vi "Func-엑셀 데이터를 그래프로 출력.vi"() -> ()   [LabVIEW 2015] (continued)
\n85\t85\t83.883\n85\t85\t83.891\n85\t85\t83.897\n85\t85\t83.907\n85\t85\t83.917\n85\t85\t83.924\n85\t85\t83.937\n85\t85\t83.942\n85\t85\t83.946\n85\t85\t83.956\n85\t85\t83.957\n85\t85.01\t83.959\n85\t85.01\t83.961\n85\t85.01\t83.965\n85\t85.01\t83.97\n85\t85.01\t83.974\n85\t85.01\t83.984\n85\t85.01\t83.996\n85\t85.01\t84\n85\t85.01\t84.004\n85\t85.01\t84.016\n85\t85.01\t84.023\n85\t85.01\t84.028\n85\t85.01\t84.036\n85\t85.01\t84.041\n85\t85.01\t84.044\n85\t85.01\t84.05\n85\t85.01\t84.058\n85\t85.01\t84.063\n85\t85.01\t84.074\n85\t85.01\t84.08\n85\t85.01\t84.095\n85\t85.01\t84.101\n85\t85.01\t84.103\n85\t85.01\t84.113\n85\t85.01\t84.116\n85\t85.01\t84.121\n85\t85.01\t84.126\n85\t85.01\t84.13\n85\t85.01\t84.139\n85\t85.01\t84.14\n85\t85.01\t84.146\n85\t85.01\t84.151\n85\t85.01\t84.157\n85\t85.01\t84.165\n85\t85.01\t84.17\n85\t85.01\t84.18\n85\t85.01\t84.185\n85\t85.01\t84.195\n85\t85.01\t84.2\n85\t85.01\t84.202\n85\t85.01\t84.207\n85\t85.01\t84.211\n85\t85.01\t84.218\n85\t85.01\t84.225\n85\t85.01\t84.23\n85\t85.01\t84.238\n85\t85.01\t84.242\n85\t85.01\t84.247\n85\t85.01\t84.253\n85\t85.01\t84.257\n85\t85.01\t84.261\n85\t85.01\t84.266\n85\t85.01\t84.273\n85\t85.01\t84.276\n85\t85.01\t84.28\n85\t85.01\t84.286\n85\t85.01\t84.292\n85\t85.01\t84.3\n85\t85.01\t84.303\n85\t85.01\t84.312\n85\t85.01\t84.321\n85\t85.01\t84.327\n85\t85.01\t84.332\n85\t85\t84.339\n85\t85\t84.35\n85\t85\t84.354\n85\t85\t84.359\n85\t85\t84.36\n85\t85\t84.367\n85\t85\t84.372\n85\t85\t84.376\n85\t85\t84.385\n85\t85\t84.395\n85\t85\t84.406\n85\t85\t84.411\n85\t85\t84.419\n85\t85\t84.423\n85\t85\t84.432\n85\t85\t84.433\n85\t85\t84.438\n85\t85\t84.446\n85\t85\t84.448\n85\t85\t84.454\n85\t85\t84.46\n85\t85\t84.464\n85\t85\t84.47\n85\t85\t84.474\n85\t85\t84.48\n85\t85\t84.484\n85\t85\t84.487\n85\t85\t84.494\n85\t85\t84.5\n85\t85\t84.507\n85\t85\t84.516\n85\t85\t84.524\n85\t85\t84.53\n85\t85\t84.536\n85\t85\t84.544\n85\t85\t84.547\n85\t85\t84.552\n85\t85\t84.556\n85\t85\t84.564\n85\t85\t84.569\n85\t85\t84.575\n85\t85\t84.582\n85\t85\t84.59\n85\t85\t84.595\n85\t85\t84.595\n85\t85\t84.602\n85\t85\t84.605\n85\t85\t84.61\n85\t85\t84.614\n85\t85\t84.62\n85\t85\t84.626\n85\t85\t84.634\n85\t85\t84.636\n85\t85\t84.64\n85\t85\t84.642\n85\t85\t84.648\n85\t85\t84.658\n85\t85\t84.659\n85\t85\t84.665\n85\t85\t84.671\n85\t85\t84.679\n85\t85\t84.684\n85\t85\t84.692\n85\t85\t84.699\n85\t85\t84.705\n85\t85\t84.715\n85\t85\t84.715\n85\t85\t84.72\n85\t85\t84.729\n85\t85\t84.736\n85\t85\t84.745\n85\t85\t84.751\n85\t85\t84.759\n85\t85\t84.764\n85\t85\t84.769\n85\t85\t84.773\n85\t85\t84.782\n85\t85\t84.787\n85\t85\t84.791\n85\t85\t84.804\n85\t85\t84.804\n85\t85\t84.81\n85\t85\t84.812\n85\t85\t84.818\n85\t85\t84.823\n85\t85\t84.823\n85\t85\t84.83\n85\t85\t84.833\n85\t85\t84.84\n85\t85\t84.846\n85\t85\t84.854\n85\t85\t84.863\n85\t85\t84.866\n85\t85\t84.872\n85\t85\t84.878\n85\t85\t84.879\n85\t85\t84.884\n85\t85\t84.886\n85\t85\t84.891\n85\t85\t84.902\n85\t85\t84.904\n85\t85\t84.91\n85\t85\t84.92\n85\t85\t84.922\n85\t85\t84.927\n85\t85\t84.932\n85\t85\t84.939\n85\t85\t84.946\n85\t85\t84.948\n85\t85\t84.953\n85\t85\t84.961\n85\t85\t84.965\n85\t85\t84.969\n85\t85\t84.973\n85\t85\t84.979\n85\t85\t84.987\n85\t85\t84.993\n85\t85\t84.996\n85\t85\t85.003\n85\t85\t85.014\n85\t85\t85.018\n85\t85\t85.023\n85\t85\t85.032\n85\t85\t85.036\n85\t85\t85.043\n85\t85\t85.048\n85\t85\t85.053\n85\t85\t85.059\n85\t85\t85.062\n85\t85\t85.067\n85\t85\t85.068\n85\t85\t85.069\n85\t85\t85.072\n85\t85\t85.075\n85\t85\t85.079\n85\t85\t85.083\n85\t85\t85.089\n85\t85\t85.096\n85\t85\t85.104\n85\t85\t85.11\n85\t85\t85.117\n85\t85\t85.128\n85\t85\t85.136\n85\t85\t85.14\n85\t85\t85.146\n85\t85\t85.153\n85\t85\t85.155\n85\t85\t85.156\n85\t85\t85.159\n85\t85\t85.163\n85\t85\t85.169\n85\t85\t85.171\n85\t85\t85.175\n85\t85\t85.185\n85\t85\t85.189\n85\t85\t85.196\n85\t85\t85.198\n85\t85\t85.203\n85\t85\t85.21\n85\t85\t85.216\n85\t85\t85.22\n85\t85\t85.227\n85\t85\t85.238\n85\t85\t85.244\n85\t85\t85.251\n85\t85\t85.253\n85\t85\t85.257\n85\t85\t85.261\n85\t85\t85.262\n85\t85\t85.263\n85\t85\t85.268\n85\t85\t85.271\n85\t85\t85.277\n85\t85\t85.283\n85\t85\t85.287\n85\t85\t85.297\n85\t85\t85.297\n85\t85\t85.302\n85\t85\t85.309\n85\t85\t85.316\n85\t85\t85.324\n85\t85\t85.333\n85\t85\t85.343\n85\t85\t85.35\n85\t85\t85.356\n85\t85\t85.36\n85\t85\t85.367\n85\t85\t85.37\n85\t85\t85.372\n85\t85\t85.375\n85\t85\t85.377\n85\t85\t85.383\n85\t85\t85.382\n85\t85\t85.384\n85\t85\t85.384\n85\t85\t85.395\n85\t85\t85.4\n85\t85\t85.401\n85\t85\t85.408\n85\t85\t85.414\n85\t85\t85.42\n85\t85\t85.424\n85\t85\t85.432\n85\t85\t85.438\n85\t85\t85.446\n85\t85\t85.451\n85\t85\t85.455\n85\t85\t85.459\n85\t85\t85.464\n85\t85\t85.471\n85\t85\t85.48\n85\t85\t85.484\n85\t85\t85.493\n85\t85\t85.495\n85\t85\t85.495\n85\t85\t85.499\n85\t85\t85.5\n85\t85\t85.502\n85\t85\t85.508\n85\t85\t85.516\n85\t85\t85.527\n85\t85\t85.537\n85\t85\t85.542\n85\t85\t85.548\n85\t85\t85.552\n85\t85\t85.552\n85\t85\t85.555\n85\t85\t85.557\n85\t85\t85.563\n85\t85\t85.568\n85\t85\t85.573\n85\t85\t85.58\n85\t85\t85.583\n85\t85\t85.588\n85\t85\t85.591\n85\t85\t85.598\n85\t85\t85.604\n85\t85\t85.609\n85\t85\t85.616\n85\t85\t85.62\n85\t85\t85.622\n85\t85\t85.625\n85\t85\t85.632\n85\t85\t85.634\n85\t85\t85.634\n85\t85\t85.639\n85\t85\t85.643\n85\t85\t85.647\n85\t85\t85.648\n85\t85\t85.657\n85\t85\t85.666\n85\t85\t85.668\n85\t85\t85.675\n85\t85\t85.682\n85\t85\t85.685\n85\t85\t85.686\n85\t85\t85.688\n85\t85\t85.693\n85\t85\t85.7\n85\t85\t85.703\n85\t85\t85.715\n85\t85\t85.721\n85\t85\t85.724\n85\t85\t85.732\n85\t85\t85.734\n85\t85\t85.736\n85\t85\t85.738\n85\t85\t85.743\n85\t85\t85.753\n85\t85\t85.758\n85\t85\t85.762\n85\t85\t85.764\n85\t85\t85.769\n85\t85\t85.771\n85\t85\t85.774\n85\t85\t85.775\n85\t85\t85.783\n85\t85\t85.798\n85\t85\t85.802\n85\t85\t85.807\n85\t85\t85.812\n85\t85\t85.816\n85\t85\t85.819\n85\t85\t85.816\n85\t85\t85.821\n85\t85\t85.829\n85\t85\t85.833\n85\t85\t85.834\n85\t85\t85.839\n85\t85\t85.848\n85\t85\t85.853\n85\t85\t85.854\n85\t85\t85.858\n85\t85\t85.868\n85\t85\t85.871\n85\t85\t85.872\n85\t85\t85.874\n85\t85\t85.885\n85\t85\t85.89\n85\t85\t85.895\n85\t85\t85.9\n85\t85\t85.904\n85\t85\t85.909\n85\t85\t85.912\n85\t85\t85.916\n85\t85\t85.918\n85\t85\t85.925\n85\t85\t85.93\n85\t85\t85.938\n85\t85\t85.942\n85\t85\t85.944\n85\t85\t85.953\n85\t85\t85.953\n85\t85\t85.955\n85\t85\t85.96\n85\t85\t85.964\n85\t85\t85.965\n85\t85\t85.973\n85\t85\t85.978\n85\t85\t85.98\n85\t85\t85.983\n85\t85\t85.986\n85\t85\t85.991\n85\t85\t85.994\n85\t85\t85.995\n85\t85\t86.002\n85\t85\t86.005\n85\t85\t86.012\n85\t85\t86.02\n85\t85\t86.024\n85\t85\t86.028\n85\t85\t86.03\n85\t85\t86.032\n85\t85\t86.037\n85\t85\t86.039\n85\t85\t86.04\n85\t85\t86.046\n85\t85\t86.049\n85\t85\t86.054\n85\t85\t86.058\n85\t85\t86.061\n85\t85\t86.066\n85\t85\t86.072\n85\t85\t86.079\n85\t85\t86.087\n85\t85\t86.091\n85\t85\t86.096\n85\t85\t86.098\n85\t85\t86.102\n85\t85\t86.109\n85\t85\t86.113\n85\t85\t86.118\n85\t85\t86.117\n85\t85\t86.122\n85\t85\t86.123\n85\t85\t86.128\n85\t85\t86.134\n85\t85\t86.138\n85\t85\t86.146\n85\t85\t86.151\n85\t85\t86.159\n85\t85\t86.159\n85\t85\t86.166\n85\t85\t86.167\n85\t85\t86.171\n85\t85.01\t86.178\n85\t85.01\t86.176\n85\t85.01\t86.182\n85\t85.01\t86.187\n85\t85.01\t86.193\n85\t85.01\t86.196\n85\t85.01\t86.2\n85\t85.01\t86.205\n85\t85.01\t86.204\n85\t85.01\t86.208\n85\t85.01\t86.214\n85\t85.01\t86.222\n85\t85.01\t86.227\n85\t85.01\t86.232\n85\t85.01\t86.236\n85\t85.01\t86.239\n85\t85.01\t86.239\n85\t85.01\t86.24\n85\t85.01\t86.238\n85\t85.01\t86.245\n85\t85.01\t86.249\n85\t85.01\t86.252\n85\t85.01\t86.253\n85\t85.01\t86.259\n85\t85.01\t86.266\n85\t85.01\t86.27\n85\t85.01\t86.275\n85\t85.01\t86.279\n85\t85.01\t86.287\n85\t85.01\t86.289\n85\t85.01\t86.29\n85\t85.01\t86.293\n85\t85.01\t86.293\n85\t85.01\t86.301\n85\t85.01\t86.304\n85\t85.01\t86.308\n85\t85.01\t86.317\n85\t85.01\t86.326\n85\t85.01\t86.328\n85\t85.01\t86.331\n85\t85.01\t86.334\n85\t85.01\t86.34\n85\t85.01\t86.342\n85\t85.01\t86.343\n85\t85.01\t86.349\n85\t85.01\t86.355\n85\t85.01\t86.36\n85\t85\t86.364\n85\t85\t86.37\n85\t85.01\t86.373\n85\t85.01\t86.379\n85\t85.01\t86.382\n85\t85.01\t86.383\n85\t85.01\t86.389\n85\t85.01\t86.393\n85\t85\t86.398\n85\t85.01\t86.404\n85\t85.01\t86.407\n85\t85.01\t86.411\n85\t85.01\t86.413\n85\t85.01\t86.411\n85\t85.01\t86.412\n85\t85.01\t86.416\n85\t85\t86.419\n85\t85\t86.423\n85\t85\t86.429\n85\t85\t86.436\n85\t85\t86.438\n85\t85\t86.441\n85\t85\t86.445\n85\t85\t86.448\n85\t85\t86.452\n85\t85\t86.458\n85\t85\t86.469\n85\t85\t86.472\n85\t85\t86.477\n85\t85\t86.484\n85\t85\t86.484\n85\t85\t86.485\n85\t85\t86.487\n85\t85\t86.489\n85\t85\t86.495\n85\t85\t86.499\n85\t85\t86.501\n85\t85\t86.501\n85\t85\t86.504\n85\t85\t86.507\n85\t85\t86.512\n85\t85\t86.516\n85\t85\t86.523\n85\t85\t86.531\n85\t85\t86.536\n85\t85\t86.54\n85\t85\t86.545\n85\t85\t86.549\n85\t85\t86.55\n85\t85\t86.556\n85\t85\t86.561\n85\t85\t86.565\n85\t85\t86.566\n85\t85\t86.568\n85\t85\t86.575\n85\t85\t86.575\n85\t85\t86.579\n85\t85\t86.583\n85\t85\t86.588\n85\t85\t86.593\n85\t85\t86.595\n85\t85\t86.601\n85\t85\t86.604\n85\t85\t86.609\n85\t85\t86.611\n85\t85\t86.618\n85\t85\t86.623\n85\t85\t86.628\n85\t85\t86.629\n85\t85\t86.635\n85\t85\t86.639\n85\t85\t86.637\n85\t85\t86.637\n85\t85\t86.638\n85\t85\t86.641\n85\t85\t86.643\n85\t85\t86.647\n85\t85\t86.651\n85\t85\t86.656\n85\t85\t86.658\n85\t85\t86.665\n85\t85\t86.669\n85\t85\t86.677\n85\t85\t86.682\n85\t85\t86.683\n85\t85\t86.689\n85\t85\t86.693\n85\t85\t86.694\n85\t85\t86.694\n85\t85\t86.695\n85\t85\t86.699\n85\t85\t86.702\n85\t85\t86.705\n85\t85\t86.71\n85\t85\t86.713\n85\t85\t86.714\n85\t85\t86.72\n85\t85\t86.722\n85\t85\t86.727\n85\t85\t86.729\n85\t85\t86.739\n85\t85\t86.746\n85\t85\t86.75\n85\t85\t86.755\n85\t85\t86.757\n85\t85\t86.761\n85\t85\t86.766\n85\t85\t86.765\n85\t85\t86.772\n85\t85\t86.774\n85\t85\t86.775\n85\t85\t86.781\n85\t85\t86.78\n85\t85\t86.789\n85\t85\t86.79\n85\t85\t86.793\n85\t85\t86.799\n85\t85\t86.803\n85\t85\t86.805\n85\t85\t86.806\n85\t85\t86.809\n85\t85\t86.813\n85\t85\t86.816\n85\t85\t86.816\n85\t85\t86.818\n85\t85\t86.821\n85\t85\t86.825\n85\t85\t86.825\n85\t85\t86.832\n85\t85\t86.836\n85\t85\t86.842\n85\t85\t86.85\n85\t85\t86.851\n85\t85\t86.855\n85\t85\t86.854\n85\t85\t86.855\n85\t85\t86.859\n85\t85\t86.859\n85\t85\t86.865\n85\t85\t86.873\n85\t85\t86.878\n85\t85\t86.882\n85\t85\t86.887\n85\t85\t86.889\n85\t85\t86.892\n85\t85\t86.892\n85\t85\t86.893\n85\t85\t86.9\n85\t85\t86.902\n85\t85\t86.907\n85\t85\t86.907\n85\t85\t86.909\n85\t85\t86.912\n85\t85\t86.915\n85\t85\t86.917\n85\t85\t86.919\n85\t85\t86.922\n85\t85\t86.925\n85\t85\t86.933\n85\t85\t86.937\n85\t85\t86.941\n85\t85\t86.941\n85\t85\t86.953\n85\t85\t86.956\n85\t85\t86.954\n85\t85\t86.961\n85\t85\t86.964\n85\t85\t86.965\n85\t85\t86.963\n85\t85\t86.968\n85\t85\t86.973\n85\t85\t86.977\n85\t85\t86.976\n85\t85\t86.984\n85\t85\t86.988\n85\t85\t86.993\n85\t85\t86.999\n85\t85\t86.997\n85\t85\t87.004\n85\t85\t87.005\n85\t85\t87.007\n85\t85\t87.008\n85\t85\t87.013\n85\t85\t87.017\n85\t85\t87.022\n85\t85\t87.027\n85\t85\t87.029\n85\t85\t87.029\n85\t85\t87.032\n85\t85\t87.037\n85\t85\t87.041\n85\t85\t87.044\n85\t85\t87.048\n85\t85\t87.055\n85\t85\t87.058\n85\t85\t87.058\n85\t85\t87.059\n85\t85\t87.059\n85\t85\t87.065\n85\t85\t87.069\n85\t85\t87.073\n85\t85\t87.078\n85\t85\t87.085\n85\t85\t87.09\n85\t85\t87.088\n85\t85\t87.089\n85\t85\t87.091\n85\t85\t87.098\n85\t85\t87.101\n85\t85\t87.1\n85\t85\t87.106\n85\t85\t87.107\n85\t85\t87.11\n85\t85\t87.111\n85\t85\t87.112\n85\t85\t87.115\n85\t85\t87.121\n85\t85\t87.123\n85\t85\t87.128\n85\t85\t87.133\n85\t85\t87.134\n85\t85\t87.138\n85\t85\t87.142\n85\t85\t87.146\n85\t85\t87.15\n85\t85\t87.151\n85\t85\t87.156\n85\t85\t87.16\n85\t85\t87.164\n85\t85\t87.166\n85\t85\t87.166\n85\t85\t87.172\n85\t85\t87.173\n85\t85\t87.172\n85\t85\t87.172\n85\t85\t87.172\n85\t85\t87.179\n85\t85\t87.18\n85\t85\t87.19\n85\t85\t87.196\n85\t85\t87.2\n85\t85\t87.208\n85\t85\t87.21\n85\t85\t87.212\n85\t85\t87.213\n85\t85\t87.214\n85\t85\t87.218\n85\t85\t87.223\n85\t85\t87.226\n85\t85\t87.226\n85\t85\t87.227\n85\t85\t87.231\n85\t85\t87.236\n85\t85\t87.237\n85\t85\t87.239\n85\t85\t87.241\n85\t85\t87.245\n85\t85\t87.245\n85\t85\t87.244\n85\t85\t87.248\n85\t85\t87.252\n85\t85\t87.258\n85\t85\t87.26\n85\t85\t87.265\n85\t85\t87.27\n85\t85\t87.269\n85\t85\t87.274\n85\t85\t87.281\n85\t85\t87.285\n85\t85\t87.289\n85\t85\t87.289\n85\t85\t87.292\n85\t85\t87.288\n85\t85\t87.294\n85\t85\t87.297\n85\t85\t87.303\n85\t85\t87.305\n85\t85\t87.308\n85\t85\t87.311\n85\t85\t87.31\n85\t85\t87.307\n85\t85\t87.311\n85\t85\t87.313\n85\t85\t87.316\n85\t85\t87.319\n85\t85\t87.321\n85\t85\t87.329\n85\t85\t87.328\n85\t85\t87.333\n85\t85\t87.339\n85\t85\t87.345\n85\t85\t87.349\n85\t85\t87.351\n85\t85\t87.352\n85\t85\t87.355\n85\t85\t87.356\n85\t85\t87.361\n85\t85\t87.366\n85\t85\t87.366\n85\t85\t87.371\n85\t85\t87.369\n85\t85\t87.371\n85\t85\t87.377\n85\t85\t87.372\n85\t85\t87.38\n85\t85\t87.383\n85\t85\t87.388\n85\t85\t87.392\n85\t85\t87.393\n85\t85\t87.397\n85\t85\t87.399\n85\t85\t87.404\n85\t85\t87.408\n85\t85\t87.411\n85\t85\t87.41\n85\t85\t87.414\n85\t85\t87.417\n85\t85\t87.414\n85\t85\t87.419\n85\t85\t87.423\n85\t85\t87.426\n85\t85\t87.427\n85\t85\t87.427\n85\t85\t87.436\n85\t85\t87.442\n85\t85\t87.442\n85\t85\t87.447\n85\t85\t87.45\n85\t85\t87.454\n85\t85\t87.454\n85\t85\t87.454\n85\t85\t87.452\n85\t85\t87.458\n85\t85\t87.462\n85\t85\t87.468\n85\t85\t87.47\n85\t85\t87.471\n85\t85\t87.479\n85\t85\t87.481\n85\t85\t87.483\n85\t85\t87.486\n85\t85\t87.485\n85\t85\t87.489\n85\t85\t87.495\n85\t85\t87.498\n85\t85\t87.498\n85\t85\t87.5\n85\t85\t87.503\n85\t85\t87.505\n85\t85\t87.507\n85\t85\t87.508\n85\t85\t87.513\n85\t85\t87.517\n85\t85\t87.519\n85\t85\t87.52\n85\t85\t87.521\n85\t85\t87.521\n85\t85\t87.523\n85\t85\t87.523\n85\t85\t87.527\n85\t85\t87.537\n85\t85\t87.542\n85\t85\t87.546\n85\t85\t87.546\n85\t85\t87.552\n85\t85\t87.554\n85\t85\t87.554\n85\t85\t87.547\n85\t85\t87.549\n85\t85\t87.552\n85\t85\t87.556\n85\t85\t87.557\n85\t85\t87.561\n85\t85\t87.571\n85\t85\t87.575\n85\t85\t87.577\n85\t85\t87.574\n85\t85\t87.577\n85\t85\t87.576\n85\t85\t87.575\n85\t85\t87.58\n85\t85\t87.584\n85\t85\t87.588\n85\t85\t87.593\n85\t85\t87.596\n85\t85\t87.595\n85\t85\t87.596\n85\t85\t87.599\n85\t85\t87.601\n85\t85\t87.602\n85\t85\t87.607\n85\t85\t87.612\n85\t85\t87.616\n85\t85\t87.618\n85\t85\t87.619\n85\t85\t87.625\n85\t85\t87.626\n85\t85\t87.631\n85\t85\t87.631\n85\t85\t87.631\n85\t85\t87.633\n85\t85\t87.636\n85\t85\t87.636\n85\t85\t87.635\n85\t85\t87.641\n85\t85\t87.643\n85\t85\t87.647\n85\t85\t87.646\n85\t85\t87.655\n85\t85\t87.66\n85\t85\t87.661\n85\t85\t87.663\n85\t85\t87.666\n85\t85\t87.668\n85\t85\t87.671\n85\t85\t87.675\n85\t85\t87.678\n85\t85\t87.68\n85\t85\t87.68\n85\t85\t87.682\n85\t85\t87.684\n85\t85\t87.683\n85\t85\t87.686\n85\t85\t87.686\n85\t85\t87.693\n85\t85\t87.698\n85\t85\t87.698\n85\t85\t87.698\n85\t85\t87.7\n85\t85\t87.703\n85\t85\t87.704\n85\t85\t87.706\n85\t85\t87.709\n85\t85\t87.72\n85\t85\t87.724\n85\t85\t87.727\n85\t85\t87.728\n85\t85\t87.73\n85\t85\t87.732\n85\t85\t87.73\n85\t85\t87.735\n85\t85\t87.739\n85\t85\t87.743\n85\t85\t87.748\n85\t85\t87.75\n85\t85\t87.754\n85\t85\t87.754\n85\t85\t87.75\n85\t85\t87.757\n85\t85\t87.757\n85\t85\t87.76\n85\t85\t87.76\n85\t85\t87.764\n85\t85\t87.77\n85\t85\t87.768\n85\t85\t87.771\n85\t85\t87.773\n85\t85\t87.777\n85\t85\t87.78\n85\t85\t87.782\n85\t85\t87.787\n85\t85\t87.788\n85\t85\t87.793\n85\t85\t87.796\n85\t85\t87.793\n85\t85\t87.799\n85\t85\t87.801\n85\t85\t87.804\n85\t85\t87.802\n85\t85\t87.803\n85\t85\t87.809\n85\t85\t87.809\n85\t85\t87.811\n85\t85\t87.81\n85\t85\t87.813\n85\t85\t87.815\n85\t85\t87.816\n85\t85\t87.817\n85\t85\t87.821\n85\t85\t87.83\n85\t85\t87.835\n85\t85\t87.838\n85\t85\t87.842\n85\t85\t87.843\n85\t85\t87.838\n85\t85\t87.842\n85\t85\t87.843\n85\t85\t87.847\n85\t85\t87.846\n85\t85\t87.852\n85\t85\t87.855\n85\t85\t87.854\n85\t85\t87.856\n85\t85\t87.857\n85\t85\t87.86\n85\t85\t87.859\n85\t85\t87.863\n85\t85\t87.867\n85\t85\t87.868\n85\t85\t87.869\n85\t85\t87.875\n85\t85\t87.878\n85\t85\t87.884\n85\t85\t87.886\n85\t85\t87.886\n85\t85\t87.886\n85\t85\t87.888\n85\t85\t87.889\n85\t85\t87.886\n85\t85\t87.888\n85\t85\t87.894\n85\t85\t87.899\n85\t85\t87.894\n85\t85\t87.897\n85\t85\t87.9\n85\t85\t87.904\n85\t85\t87.901\n85\t85\t87.902\n85\t85\t87.913\n85\t85\t87.912\n85\t85\t87.914\n85\t85\t87.917\n85\t85\t87.923\n85\t85\t87.922\n85\t85\t87.921\n85\t85\t87.929\n85\t85\t87.932\n85\t85\t87.932\n85\t85\t87.934\n85\t85\t87.937\n85\t85\t87.939\n85\t85\t87.941\n85\t85\t87.946\n85\t85\t87.95\n85\t85\t87.952\n85\t85\t87.95\n85\t85\t87.951\n85\t85\t87.951\n85\t85\t87.95\n85\t85\t87.951\n85\t85\t87.954\n85\t85\t87.963\n85\t85\t87.966\n85\t85\t87.969\n85\t85\t87.97\n85\t85\t87.97\n85\t85\t87.973\n85\t85\t87.973\n85\t85\t87.979\n85\t85\t87.986\n85\t85\t87.984\n85\t85\t87.989\n85\t85\t87.988\n85\t85\t87.989\n85\t85\t87.988\n85\t85\t87.989\n85\t85\t87.994\n85\t85\t87.993\n85\t85\t87.999\n85\t85\t88.005\n85\t85\t88.007\n85\t85\t88.007\n85\t85\t88.011\n85\t85\t88.018\n85\t85\t88.02\n85\t85\t88.015\n85\t85\t88.018\n85\t85\t88.016\n85\t85\t88.016\n85\t85\t88.017\n85\t85\t88.018\n85\t85\t88.023\n85\t85\t88.027\n85\t85\t88.037\n85\t85\t88.037\n85\t85\t88.038\n85\t85\t88.041\n85\t85\t88.044\n85\t85\t88.045\n85\t85\t88.047\n85\t85\t88.051\n85\t85\t88.054\n85\t85\t88.056\n85\t85\t88.061\n85\t85\t88.062\n85\t85\t88.057\n85\t85\t88.059\n85\t85\t88.059\n85\t85\t88.062\n85\t85\t88.061\n85\t85\t88.066\n85\t85\t88.072\n85\t85\t88.077\n85\t85\t88.082\n85\t85\t88.084\n85\t85\t88.085\n85\t85\t88.084\n85\t85\t88.085\n85\t85\t88.086\n85\t85\t88.085\n85\t85\t88.085\n85\t85\t88.088\n85\t85\t88.091\n85\t85\t88.092\n85\t85\t88.095\n85\t85\t88.097\n85\t85\t88.103\n85\t85\t88.103\n85\t85\t88.104\n85\t85\t88.107\n85\t85\t88.108\n85\t85\t88.107\n85\t85\t88.106\n85\t85\t88.111\n85\t85\t88.116\n85\t85\t88.115\n85\t85\t88.115\n85\t85\t88.118\n85\t85\t88.123\n85\t85\t88.123\n85\t85\t88.118\n85\t85\t88.121\n85\t85\t88.123\n85\t85\t88.123\n85\t85\t88.12\n85\t85\t88.123\n85\t85\t88.13\n85\t85\t88.133\n85\t85\t88.136\n85\t85\t88.142\n85\t85\t88.144\n85\t85\t88.143\n85\t85\t88.143\n85\t85\t88.144\n85\t85\t88.146\n85\t85\t88.144\n85\t85\t88.149\n85\t85\t88.154\n85\t85\t88.155\n85\t85\t88.158\n85\t85\t88.157\n85\t85\t88.162\n85\t85\t88.166\n85\t85\t88.165\n85\t85\t88.166\n85\t85\t88.167\n85\t85\t88.173\n85\t85\t88.171\n85\t85\t88.174\n85\t85\t88.176\n85\t85\t88.177\n85\t85\t88.18\n85\t85\t88.18\n85\t85\t88.186\n85\t85\t88.188\n85\t85\t88.187\n85\t85\t88.188\n85\t85\t88.192\n85\t85\t88.195\n85\t85\t88.196\n85\t85\t88.195\n85\t85\t88.198\n85\t85\t88.206\n85\t85\t88.206\n85\t85\t88.205\n85\t85\t88.207\n85\t85\t88.21\n85\t85\t88.215\n85\t85\t88.217\n85\t85\t88.219\n85\t85\t88.221\n85\t85\t88.225\n85\t85\t88.228\n85\t85\t88.225\n85\t85\t88.229\n85\t85\t88.23\n85\t85\t88.234\n85\t85\t88.232\n85\t85\t88.233\n85\t85\t88.234\n85\t85\t88.232\n85\t85\t88.235\n85\t85\t88.234\n85\t85\t88.238\n85\t85\t88.237\n85\t85\t88.238\n85\t85\t88.239\n85\t85\t88.241\n85\t85\t88.245\n85\t85\t88.249\n85\t85\t88.252\n85\t85\t88.255\n85\t85\t88.257\n85\t85\t88.259\n85\t85\t88.256\n85\t85\t88.25\n85\t85\t88.253\n85\t85\t88.258\n85\t85\t88.26\n85\t85\t88.263\n85\t85\t88.266\n85\t85\t88.27\n85\t85\t88.275\n85\t85\t88.273\n85\t85\t88.275\n85\t85\t88.276\n85\t85\t88.277\n85\t85\t88.281\n85\t85\t88.284\n85\t85\t88.286\n85\t85\t88.286\n85\t85\t88.29\n85\t85\t88.292\n85\t85\t88.293\n85\t85\t88.295\n85\t85\t88.298\n85\t85\t88.303\n85\t85\t88.303\n85\t85\t88.304\n85\t85\t88.305\n85\t85\t88.303\n85\t85\t88.307\n85\t85\t88.304\n85\t85\t88.303\n85\t85\t88.306\n85\t85\t88.309\n85\t85\t88.312\n85\t85\t88.311\n85\t85\t88.317\n85\t85\t88.322\n85\t85\t88.327\n85\t85\t88.33\n85\t85\t88.332\n85\t85\t88.335\n85\t85\t88.333\n85\t85\t88.332\n85\t85\t88.329\n85\t85\t88.327\n85\t85\t88.33\n85\t85\t88.33\n85\t85\t88.337\n85\t85\t88.341\n85\t85\t88.348\n85\t85\t88.35\n85\t85\t88.35\n85\t85\t88.354\n85\t85\t88.354\n85\t85\t88.354\n85\t85\t88.351\n85\t85\t88.354\n
